vi "Telnet_Read_Write.vi"(8 "error in (no error)":errorcluster, 9 "bytes to read (1024)":i32=1024, 10 "Write Telnet Command":string, 11 "connection ID":refnum<k5>) -> (2 "string out":string, 3 "connection ID out":refnum<k5>)   [LabVIEW 2018]
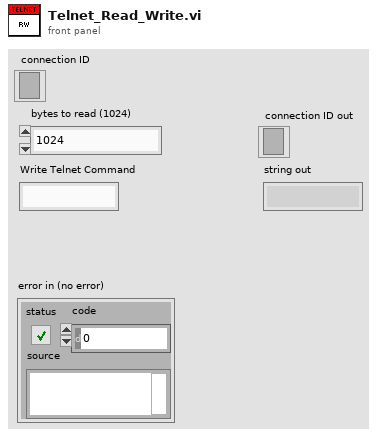
[diagram p1: front panel]
types:
  T1 = enum16{"Standard", "Buffered", "CRLF", "Immediate"}
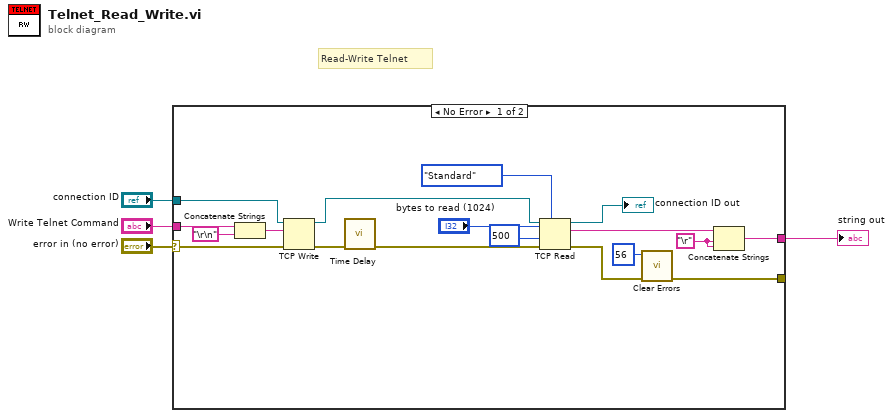
[diagram p0: block diagram]
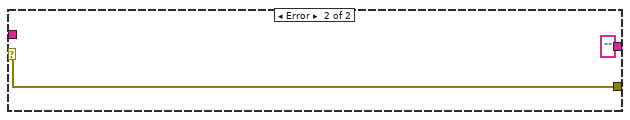
[diagram p2: hidden frame]
diagram:
  # "Read-Write Telnet"
  n1 = case shown="No Error" "error in (no error)" {
    selector: "error in (no error)" -> [w5 w23]
    tunnel: [w13 ""] -> w1
    tunnel: [w12 w23] -> _
    tunnel: "Write Telnet Command" -> [w9 _]
    tunnel: "connection ID" -> [w6 _]
    frame No Error {
      w14 = "\r"
      n2 = Concatenate Strings(w9, "\r\n") -> (w11:string)
      n3 = TCP Write(connection ID=w6, data in=w11, error in (no error)=w5) -> (connection ID out=w8:refnum<k5>, error out=w7:errorcluster)  [unwired: 1 in, 1 out]
      n4 = call "Time Delay"("error in (no error)"=w7) -> ("error out"=w16:errorcluster)  [unwired: 10 in]
      n5 = TCP Read(connection ID=w8, bytes to read="bytes to read (1024)", error in (no error)=w16, 7:T1."Standard" ("mode (standard)"), 9:500 ("timeout ms (25000)")) -> (connection ID out=→"connection ID out":refnum<k5>, data out=w15:string, error out=w19:errorcluster)
      n6 = call "Clear Errors.vi"("error in (no error)"=w19, "specific error code to clear (0: all)"=56) -> ("error out"=w12:errorcluster)  [unwired: 4 in, 1 out]
      n7 = Concatenate Strings(w15, w14, w14) -> (w13:string)
    }
    frame Error {
    }
  }
  "string out" <- w1
